vi "Enqueue.vi"(8 "error in (no error)":errorcluster, 9 "Dato":variant, 10 "Mensaje":string, 11 "Queue in":refnum<queue>) -> (0 "error out":errorcluster)   [LabVIEW 2018, in "Mensajes.lvlib"]
uses:
  Mensajes.lvlib
  Controles/Mensaje Data.ctl
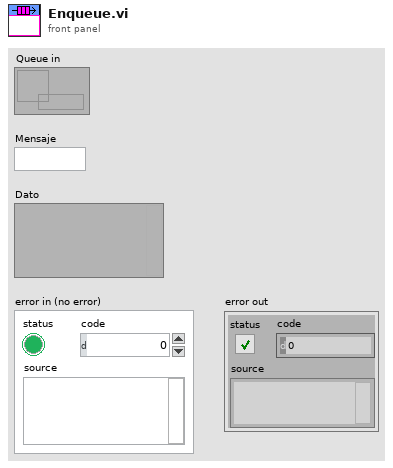
[diagram p1: front panel]
types:
  T1 = typedef "Mensaje Data.ctl" = cluster{"Mensaje":string, "Dato":variant}
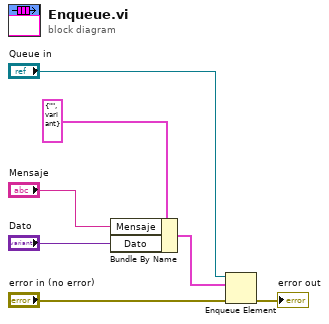
[diagram p0: block diagram]
diagram:
  n1 = Bundle By Name(cluster=T1 {"Mensaje"="", "Dato"=variant} ("element"), "Mensaje"="Mensaje", "Dato"="Dato") -> (w5:T1)
  n2 = Enqueue Element(queue="Queue in", element=w5, error in (no error)="error in (no error)") -> (error out=→"error out":errorcluster)  [unwired: 1 in, 2 out]
